vi "StartSpec.vi"(0 "Mode":T1=3 items=["Spectroscopy 1", "Spectroscopy 2", "Spectroscopy 3", "Calibration"], 1 "State":T2 items=["off", "on"], 5 "error in":T3) -> (14 "State out":T2 items=["off", "on"], 15 "Mode out":T1=3 items=["Spectroscopy 1", "Spectroscopy 2", "Spectroscopy 3", "Calibration"], 19 "error out":T3)   [LabVIEW 2016]
doc: "Activates the output and starts a spectroscopy for state = 1 and deactivates the output for state = 0 as a spectroscopy will stop autonomously."
uses:
  Controls/State_Selection.ctl
  Controls/Spectroscopy-Mode_Selection.ctl
  Controls/Error_Out.ctl
  Files_ASC500/DLL/ASC500_RemoteControlV27.dll
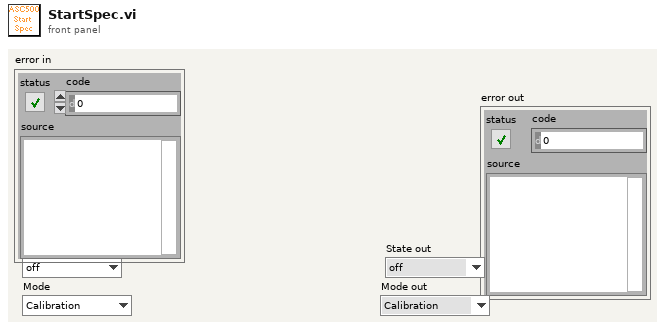
[diagram p1: front panel]
types:
  T1 = typedef "Spectroscopy-Mode_Selection.ctl" = u16
  T2 = typedef "State_Selection.ctl" = u16
  T3 = typedef "Error_Out.ctl" = errorcluster
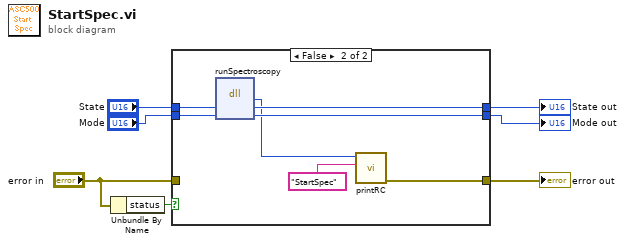
[diagram p0: block diagram]
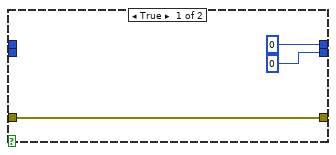
[diagram p2: hidden frame]
diagram:
  n1 = Unbundle By Name("error in") -> ("status"=w7:bool)
  n2 = case shown="False" w7 {
    tunnel: [w10 w13] -> w6
    tunnel: "State" -> [_ w17]
    tunnel: "Mode" -> [_ w16]
    tunnel: [0 ("Mode") w15] -> w3
    tunnel: [0 ("State") w14] -> w2
    tunnel: "error in" -> [w10 _]
    frame True {
    }
    frame False {
      n3 = dll-call lib="G:/SCMOperations/Share/ELE/Produkt Information/ASC500/04 Remote Control/02 development versions/2018Nov06/Files_ASC500/DLL/ASC500_RemoteControlV27.dll" fn="runSpectroscopy"("State"=w17, "Mode"=w16) -> ("return type"=w12:i32, "State"=w14:i32, "Mode"=w15:i32)  [unwired: 3 in, 2 out]
      n4 = call "printRC.vi"("additional information"="StartSpec", "RC"=w12) -> ("error out"=w13:T3)  [unwired: 9 in]
    }
  }
  "error out" <- w6
  "State out" <- w2
  "Mode out" <- w3
